vi "Rollendrehzahl (SubVI).vi"(9 "Stop":refnum<vi>, 10 "Rollendrehzahl aufzeichnen":refnum<vi>, 11 "Rollendrehzahl (Eingang)":refnum<vi>) -> ()   [LabVIEW 2014]
panel:
  in  "Export":bool
  in  "Reset Graph":bool
  in  "Aufzeichnung":bool
  out "Rollendrehzahl":dbl[](graph)
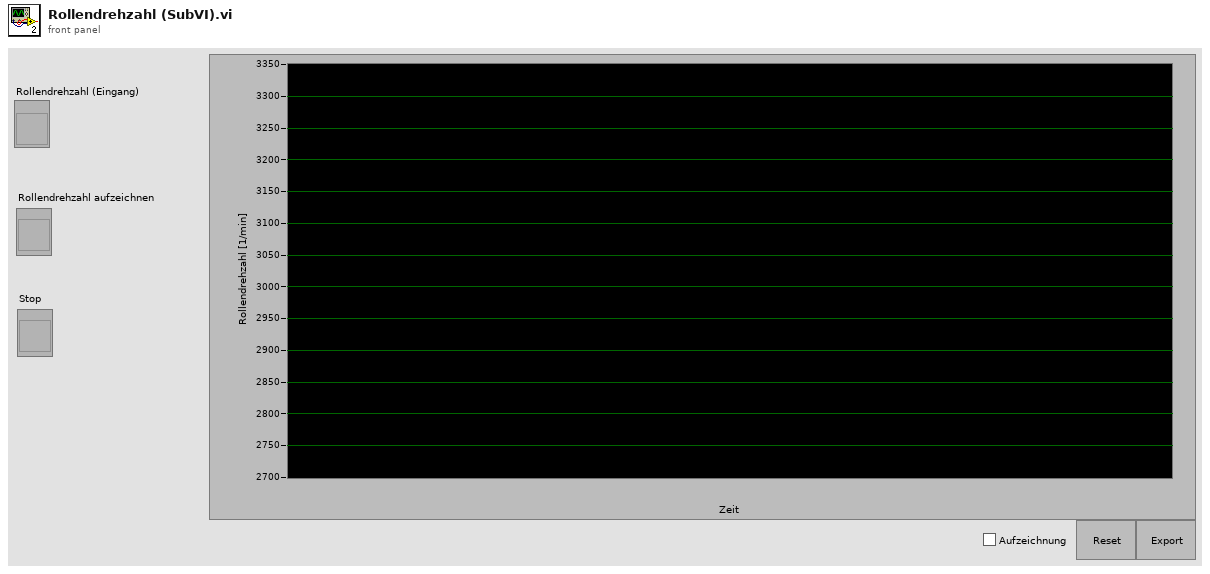
[diagram p1: front panel]
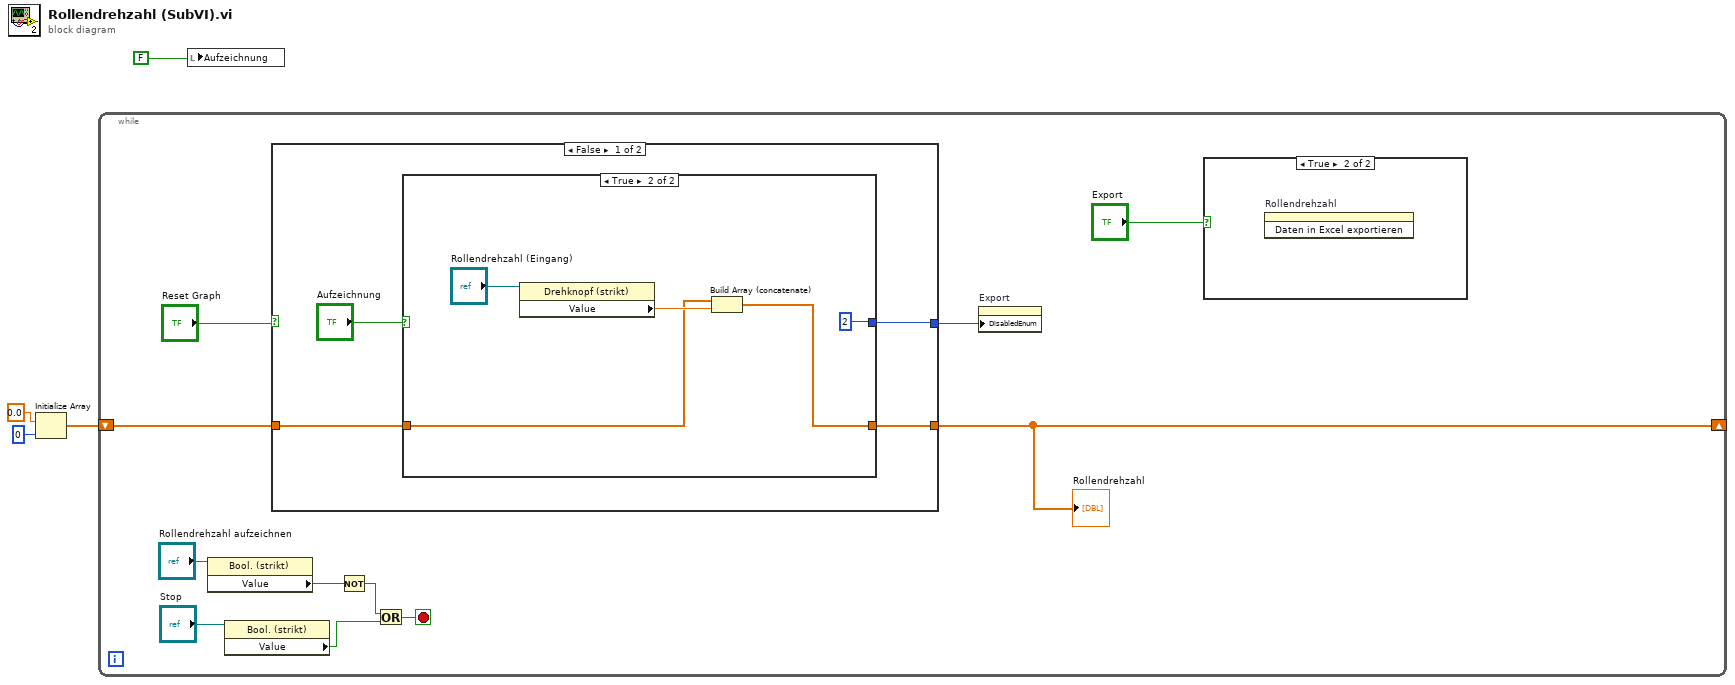
[diagram p0: block diagram]
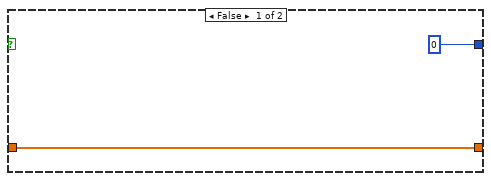
[diagram p3: hidden frame]
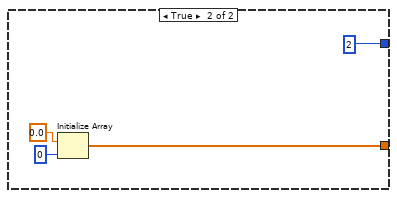
[diagram p4: hidden frame]
diagram:
  n1 = Initialize Array(0.0 ("y"), 0) -> (w2:dbl[])
  n2 = while {
    shift-right: [w10] -> _
    shift-left: w2 -> [w13]
    stop <- w8 stop-if-true
    n3 = property class="Bool. (strikt)"(reference="Rollendrehzahl aufzeichnen") -> ("Value"=w14:bool)  [unwired: 1 in, 2 out]
    n4 = property class="Bool. (strikt)"(reference="Stop") -> ("Value"=w5:bool)  [unwired: 1 in, 2 out]
    n5 = case shown="False" "Reset Graph" {
      tunnel: w13 -> [w19 _]
      tunnel: [w17 w28] -> w10
      tunnel: [w16 2] -> w11
      frame False {
        n6 = case shown="True" "Aufzeichnung" {
          tunnel: w19 -> [w21 w24]
          tunnel: [w21 w23] -> w17
          tunnel: [0 2] -> w16
          frame False {
          }
          frame True {
            n7 = property class="Drehknopf (strikt)"(reference="Rollendrehzahl (Eingang)") -> ("Value"=w26:dbl)  [unwired: 1 in, 2 out]
            n8 = Build Array (concatenate)(w24, w26) -> (w23:dbl[])
          }
        }
      }
      frame True {
        n9 = Initialize Array(0.0 ("y"), 0) -> (w28:dbl[])
      }
    }
    "Rollendrehzahl" <- w10
    n10 = Not(x=w14) -> (.not. x?=w6:bool)
    n11 = Or(x=w6, y=w5) -> (x .or. y?=w8:bool)
    n12 = property on="Export" class="Bool."("DisabledEnum"=w11) -> ()  [unwired: 2 in, 2 out]
    n13 = case shown="True" "Export" {
      frame False {
      }
      frame True {
        n14 = invoke on="Rollendrehzahl" class="SVGraph (strikt)" method="Daten in Excel exportieren"() -> ()  [unwired: 3 in, 3 out]
      }
    }
  }
  n15 = local write "Aufzeichnung"(FALSE) -> ()
